vi "FMA1600A Parse Data.vi"(7 "Error In":errorcluster, 10 "Raw FMA1600A Data":string) -> (0 "Error Out":errorcluster, 3 "FMA1600A Gas Data":T1)   [LabVIEW 2018]
uses:
  Type Definitions/FMA1600A Data.ctl
  <vilib>/Utility/error.llb/whitespace.ctl
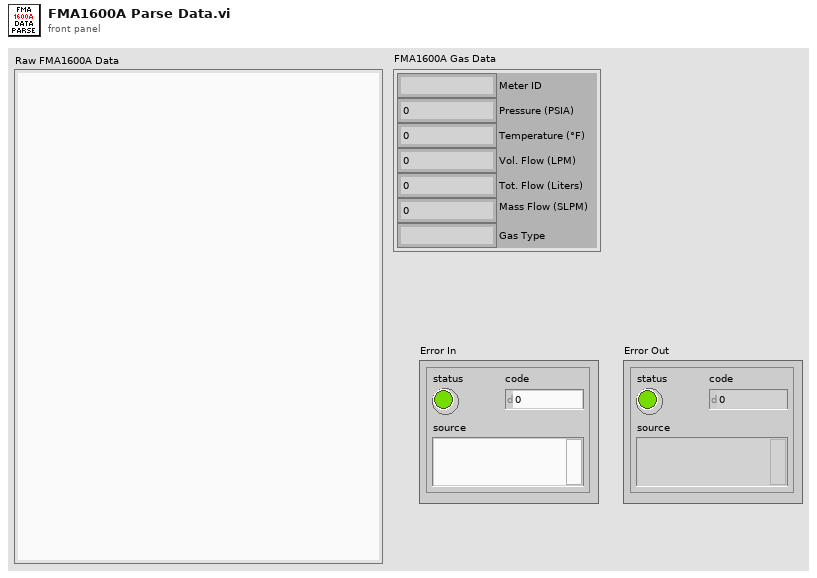
[diagram p1: front panel]
types:
  T1 = typedef "FMA1600A Data.ctl" = cluster{"Pressure (PSIA)":dbl, "Temperature (°F)":dbl, "Vol. Flow (LPM)":dbl, "Mass Flow (SLPM)":dbl, "Gas Type":string, "Tot. Flow (Liters)":dbl, "Meter ID":string}
  T2 = typedef "whitespace.ctl" = u16
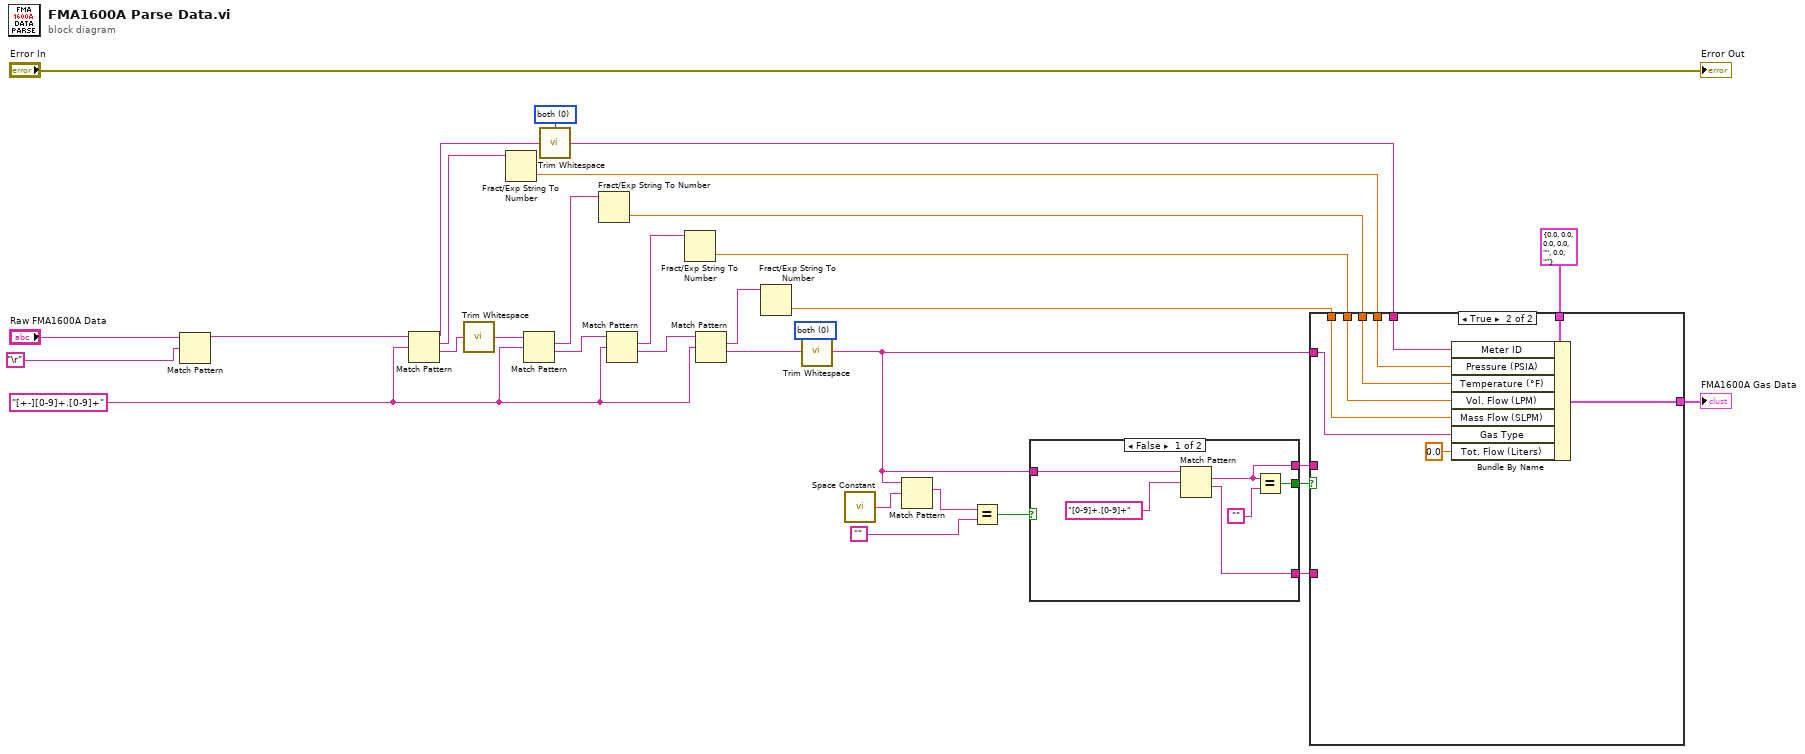
[diagram p0: block diagram]
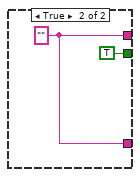
[diagram p2: hidden frame]
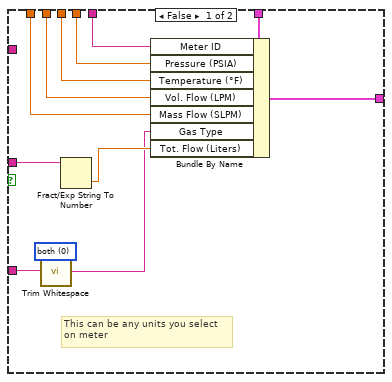
[diagram p3: hidden frame]
diagram:
  w17 = T2 0 items=["both", "start of string", "end of string"] ("location (both)")
  w28 = T2 0 items=["both", "start of string", "end of string"] ("location (both)")
  w26 = "[+-][0-9]+.[0-9]+" ("regular expression")
  n1 = Match Pattern(string="Raw FMA1600A Data", regular expression="\r") -> (before substring=w19:string)  [unwired: 1 in, 3 out]
  n2 = Match Pattern(string=w19, regular expression=w26) -> (before substring=w18:string, match substring=w29:string, after substring=w23:string)  [unwired: 1 in, 1 out]
  n3 = call <vilib>:"Trim Whitespace.vi"("string"=w23) -> ("trimmed string"=w24:string)  [unwired: 1 in]
  n4 = Fract/Exp String To Number(string=w29) -> (number=w11:dbl)  [unwired: 3 in, 1 out]
  n5 = Match Pattern(string=w24, regular expression=w26) -> (match substring=w30:string, after substring=w25:string)  [unwired: 1 in, 2 out]
  n6 = call <vilib>:"Trim Whitespace.vi"("string"=w18, "location (both)"=w17) -> ("trimmed string"=w10:string)
  n7 = Fract/Exp String To Number(string=w30) -> (number=w12:dbl)  [unwired: 3 in, 1 out]
  n8 = Match Pattern(string=w25, regular expression=w26) -> (match substring=w32:string, after substring=w16:string)  [unwired: 1 in, 2 out]
  n9 = Fract/Exp String To Number(string=w32) -> (number=w13:dbl)  [unwired: 3 in, 1 out]
  n10 = Match Pattern(string=w16, regular expression=w26) -> (match substring=w31:string, after substring=w27:string)  [unwired: 1 in, 2 out]
  n11 = Fract/Exp String To Number(string=w31) -> (number=w14:dbl)  [unwired: 3 in, 1 out]
  n12 = call <vilib>:"Trim Whitespace.vi"("string"=w27, "location (both)"=w28) -> ("trimmed string"=w5:string)
  n13 = call <vilib>:"Space Constant.vi"() -> ("String"=w1:string)
  n14 = Match Pattern(string=w5, regular expression=w1) -> (match substring=w3:string)  [unwired: 1 in, 3 out]
  n15 = Equal?(x=w3, y="") -> (x = y?=w2:bool)
  n16 = case shown="False" w2 {
    tunnel: [w37 TRUE] -> w15
    tunnel: [w35 w39] -> w7
    tunnel: [w34 w39] -> w6
    tunnel: w5 -> [w33 _]
    frame False {
      n17 = Match Pattern(string=w33, regular expression="[0-9]+.[0-9]+") -> (match substring=w35:string, after substring=w34:string)  [unwired: 1 in, 2 out]
      n18 = Equal?(x=w35, y="") -> (x = y?=w37:bool)
    }
    frame True {
      w39 = "" ("trimmed string")
    }
  }
  n19 = case shown="True" w15 {
    tunnel: w5 -> [_ w61]
    tunnel: w14 -> [w46 w60]
    tunnel: w13 -> [w47 w59]
    tunnel: w12 -> [w48 w58]
    tunnel: w11 -> [w49 w57]
    tunnel: w10 -> [w50 w56]
    tunnel: T1 {"Pressure (PSIA)"=0.0, "Temperature (°F)"=0.0, "Vol. Flow (LPM)"=0.0, "Mass Flow (SLPM)"=0.0, "Gas Type"="", "Tot. Flow (Liters)"=0.0, "Meter ID"=""} ("FMA1600A Gas Data") -> [w52 w55]
    tunnel: [w51 w54] -> w8
    tunnel: w7 -> [w44 _]
    tunnel: w6 -> [w42 _]
    frame False {
      w43 = T2 0 items=["both", "start of string", "end of string"] ("location (both)")
      # "This can be any units you select\non meter"
      n20 = call <vilib>:"Trim Whitespace.vi"("string"=w42, "location (both)"=w43) -> ("trimmed string"=w41:string)
      n21 = Fract/Exp String To Number(string=w44) -> (number=w45:dbl)  [unwired: 3 in, 1 out]
      n22 = Bundle By Name(cluster=w52, "Meter ID"=w50, "Pressure (PSIA)"=w49, "Temperature (°F)"=w48, "Vol. Flow (LPM)"=w47, "Mass Flow (SLPM)"=w46, "Gas Type"=w41, "Tot. Flow (Liters)"=w45) -> (w51:T1)
    }
    frame True {
      n23 = Bundle By Name(cluster=w55, "Meter ID"=w56, "Pressure (PSIA)"=w57, "Temperature (°F)"=w58, "Vol. Flow (LPM)"=w59, "Mass Flow (SLPM)"=w60, "Gas Type"=w61, "Tot. Flow (Liters)"=0.0) -> (w54:T1)
    }
  }
  "FMA1600A Gas Data" <- w8
  "Error Out" <- "Error In"
